vi "Get Node Reference.vi"(8 "error in":errorcluster, 11 "Node Ptr":T1 format="%.0x") -> (0 "error out":errorcluster, 1 "Base Node":refnum<k24>, 2 "BaseNodeType":refnum<k24>, 3 "Node Ptr":T1 format="%.0x")   [LabVIEW 2026, in "Template System Explorer.lvlib"]
uses:
  <vilib>/NI VeriStand/Custom Device API/Custom Device Item Ref.ctl
  NationalInstruments.VeriStand.SystemStorage
  NationalInstruments.VeriStand.SystemDefinitionAPI
  Template System Explorer.lvlib
  <vilib>/NI VeriStand/Custom Device API/Custom Device API.lvlib
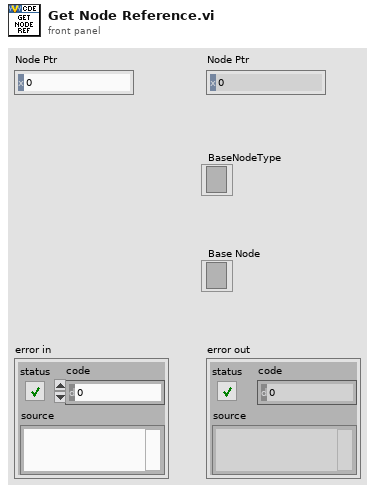
[diagram p1: front panel]
types:
  T1 = typedef "Custom Device API.lvlib/Custom Device Item Ref.ctl" = u64
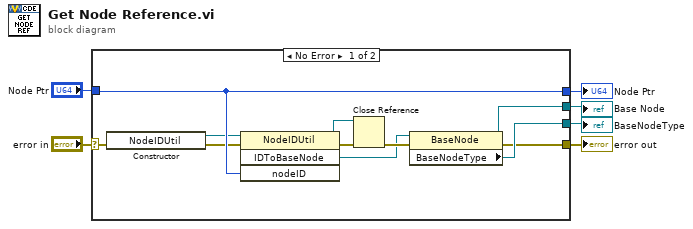
[diagram p0: block diagram]
diagram:
  n1 = case shown="No Error" "error in" {
    selector: "error in" -> [w17 w19]
    tunnel: [w9 w19] -> w5
    tunnel: [w16 _] -> w4
    tunnel: "Node Ptr" -> [w15 w18]
    tunnel: [w15 w18] -> w2
    tunnel: [w7 _] -> w1
    frame No Error {
      n2 = constructor class="NodeIDUtil"(error in=w17) -> (reference out=w10:refnum<k24>, error out=w12:errorcluster)  [unwired: 2 in, 1 out]
      n3 = invoke class="NodeIDUtil" method="IDToBaseNode"(reference=w10, error in=w12, "nodeID"=w15) -> (reference out=w11:refnum<k24>, error out=w13:errorcluster, "IDToBaseNode"=w8:refnum<k24>)  [unwired: 1 in, 1 out]
      n4 = Close Reference(reference=w11, error in (no error)=w13) -> (error out=w14:errorcluster)
      n5 = property class="BaseNode"(reference=w8, error in=w14) -> (reference out=w7:refnum<k24>, error out=w9:errorcluster, "BaseNodeType"=w16:refnum<k24>)
    }
    frame Error {
    }
  }
  "error out" <- w5
  "BaseNodeType" <- w4
  "Node Ptr" <- w2
  "Base Node" <- w1
